vi "voorbeeld.vi"() -> ()   [LabVIEW 2014]
panel:
  in  "stop":bool
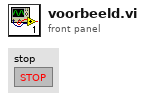
[diagram p1: front panel]
types:
  T1 = cluster{"Amplitude":dynamicdata, "Frequency":dynamicdata, "Phase":dynamicdata}
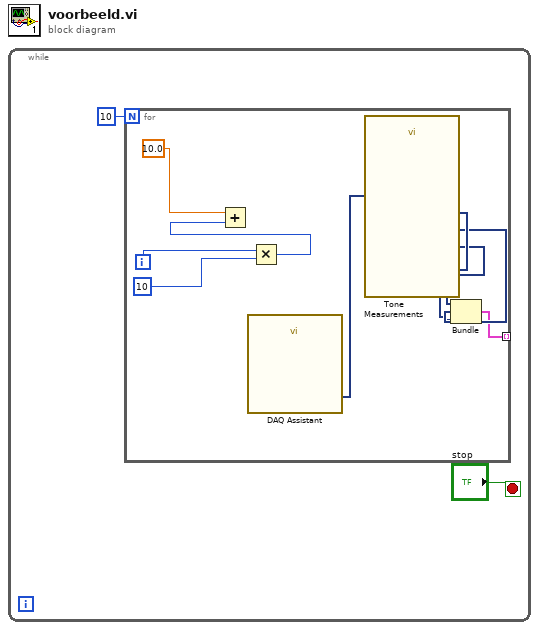
[diagram p0: block diagram]
diagram:
  n1 = while {
    stop <- "stop" stop-if-true
    n2 = for {
      N: 10 -> [_]
      tunnel: [w4] -> _ mode=indexing
      i -> [w10]
      n3 = call "DAQ Assistant"() -> ("data"=w8:dynamicdata)  [unwired: 16 in, 3 out]
      n4 = Multiply(x=w10, y=10) -> (x*y=w3:i32)
      n5 = Add(x=10.0 ("Frequency"), y=w3) -> ()  [unwired: 1 out]
      n6 = call "Tone Measurements"("Signals"=w8) -> ("Phase"=w5:dynamicdata, "Frequency"=w6:dynamicdata, "Amplitude"=w7:dynamicdata)  [unwired: 7 in, 1 out]
      n7 = Bundle("Amplitude"=w7, "Frequency"=w6, "Phase"=w5) -> (w4:T1)  [unwired: 1 in]
    }
  }
